vi "Log Clear.vi"   [LabVIEW 2014]
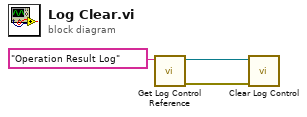
[diagram p0: block diagram]
diagram:
  n1 = call "Get Log Control Reference.vi"("Log Control  Name"="Operation Result Log") -> ("エラー出力"=w1:errorcluster, "Referece to Log Control"=w2:refnum<vi>)  [unwired: 9 in]
  n2 = call "Clear Log Control.vi"("エラー入力 (エラーなし)"=w1, "Control“ü—Í"=w2) -> ()  [unwired: 9 in, 1 out]
